vi "STORE_FREE_INPUT.vi"(9 "CURRENT_YEAR_DATA":string, 10 "ECODE 2":string, 11 "connection reference":T1) -> ()   [LabVIEW 2015]
uses:
  <vilib>/addons/database/Connection.llb/Conn ObjectReference.ctl
  Controls/ITEM_INFORMATION_CLUSTER.ctl
  Controls/ITEM_CODE_CLUSTER.ctl
  <vilib>/addons/database/Connection.llb/Conn Execute.vi
  <vilib>/addons/database/Recordset.llb/Rec Destroy - Connection.vi
  <vilib>/addons/database/_DB Variant To Data/Database Variant To Data.xnode
  <vilib>/addons/database/NI_Database_API.lvlib
  <vilib>/addons/database/Connection.llb/DB Tools Open Connec (String).vi
panel:
  in  "Store Stock":dbl
  in  "Lot Maker":string
  out "Invoice Date":timestamp format="%<%d/%m/%Y>T"
  in  "Location":string
  in  "Maker Code":string
  in  "Invoice No.":string
  in  "BUTTON_EXIT":bool
  in  "BUTTON_INPUT":bool
  in  "Unit 2":string
  in  "Quantity":dbl
  in  "Item Code":string
  in  "QR Code (F3)":string
  in  "Maker":string
  in  "Part Name":string
  in  "Product":string
  out "ECODE":string
  out "Input Date":timestamp format="%<%d/%m/%Y>T"
  in  "Input No.(F1)":string
  # "FREE INPUT"
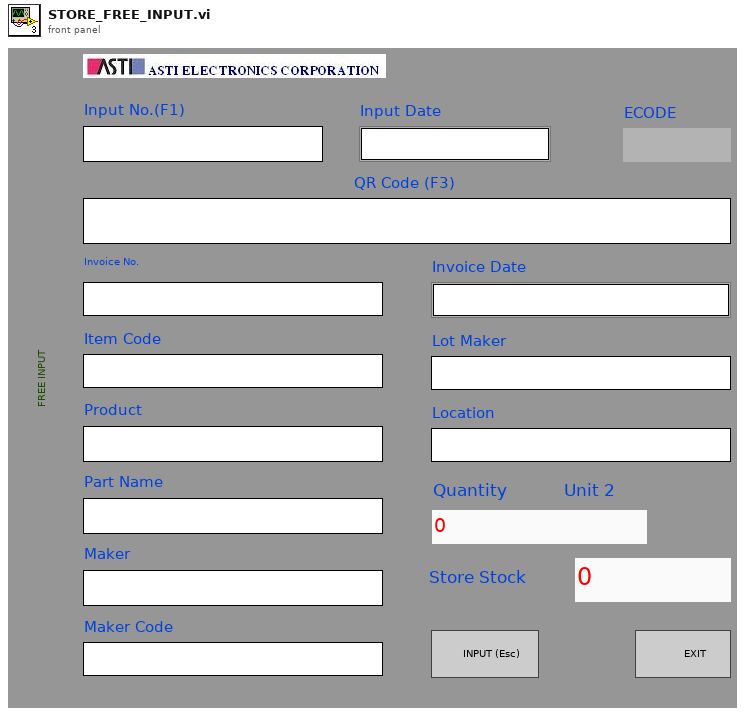
[diagram p1: front panel]
types:
  T1 = typedef "NI_Database_API.lvlib/Conn ObjectReference.ctl" = refnum<k1>
  T2 = typedef "ITEM_CODE_CLUSTER.ctl" = cluster{"ITEM_CODE":string, "INVOICE_NO":string, "INVOICE_DATE":timestamp, "LOT_MAKER":string, "QUANTITY":dbl, "INVOICE_ECODE":string, "INPUT_NO":string, "INPUT_DATE":timestamp, "INPUT_ECODE":string, "LINEBACK_NO":string, "LINEBACK_DATE":timestamp, "LINEBACK_ECODE":string, "OUTPUT_NO":string, "OUTPUT_DATE":timestamp, "OUTPUT_ECODE":string, "DESTINATION":string}
  T3 = cluster{"INVOICE_DATE":timestamp, "LOT_MAKER":string, "INVOICE_NO":string}[]
  T4 = typedef "ITEM_INFORMATION_CLUSTER.ctl" = cluster{"PRODUCT":string, "ITEM_CODE":string, "PART_NAME":string, "MAKER":string, "PART_NO":string, "LOT_SIZE":dbl, "UNIT":string, "LENGTH-OFFSET":string, "BARCODE":string, "PROCESS":string, "INVENTORY_LOCAL":string, "TARE":dbl, "SAMPLE":dbl}
  T5 = cluster{"ITEM_CODE":string, "INVOICE_NO":string, "INVOICE_DATE":timestamp, "LOT_MAKER":string, "QUANTITY":dbl, "INVOICE_ECODE":string, "INPUT_NO":string, "INPUT_DATE":timestamp, "INPUT_ECODE":string, "LINEBACK_NO":string, "LINEBACK_DATE":timestamp, "LINEBACK_ECODE":string, "OUTPUT_NO":string, "OUTPUT_DATE":timestamp, "OUTPUT_ECODE":string, "DESTINATION":string}
  T6 = cluster{"INVOICE_DATE":timestamp, "LOT_MAKER":string, "INVOICE_NO":string}
  T7 = typedef "NI_Database_API.lvlib/Rec ObjectReference.ctl" = refnum<k1>
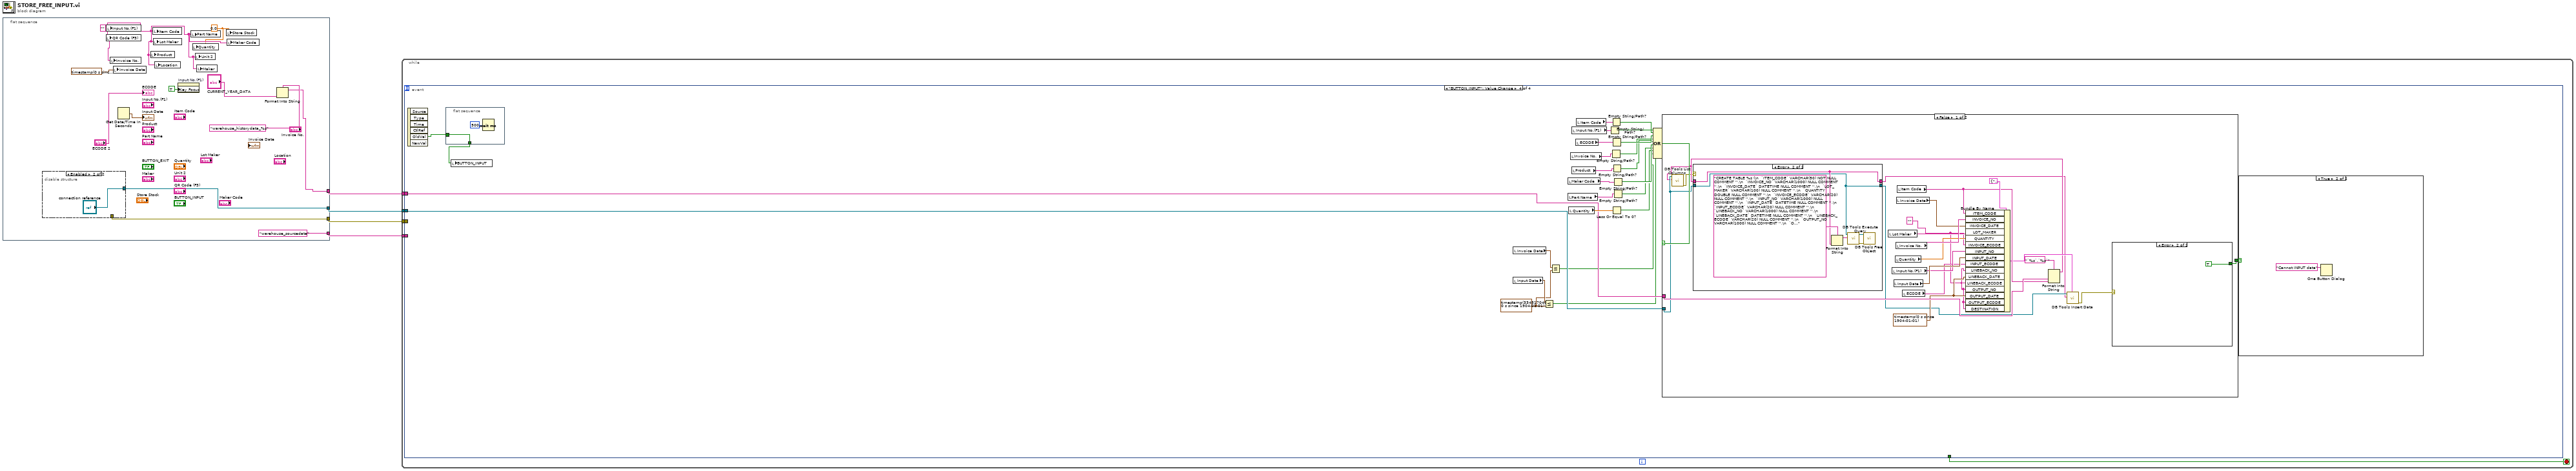
[diagram p0: block diagram]
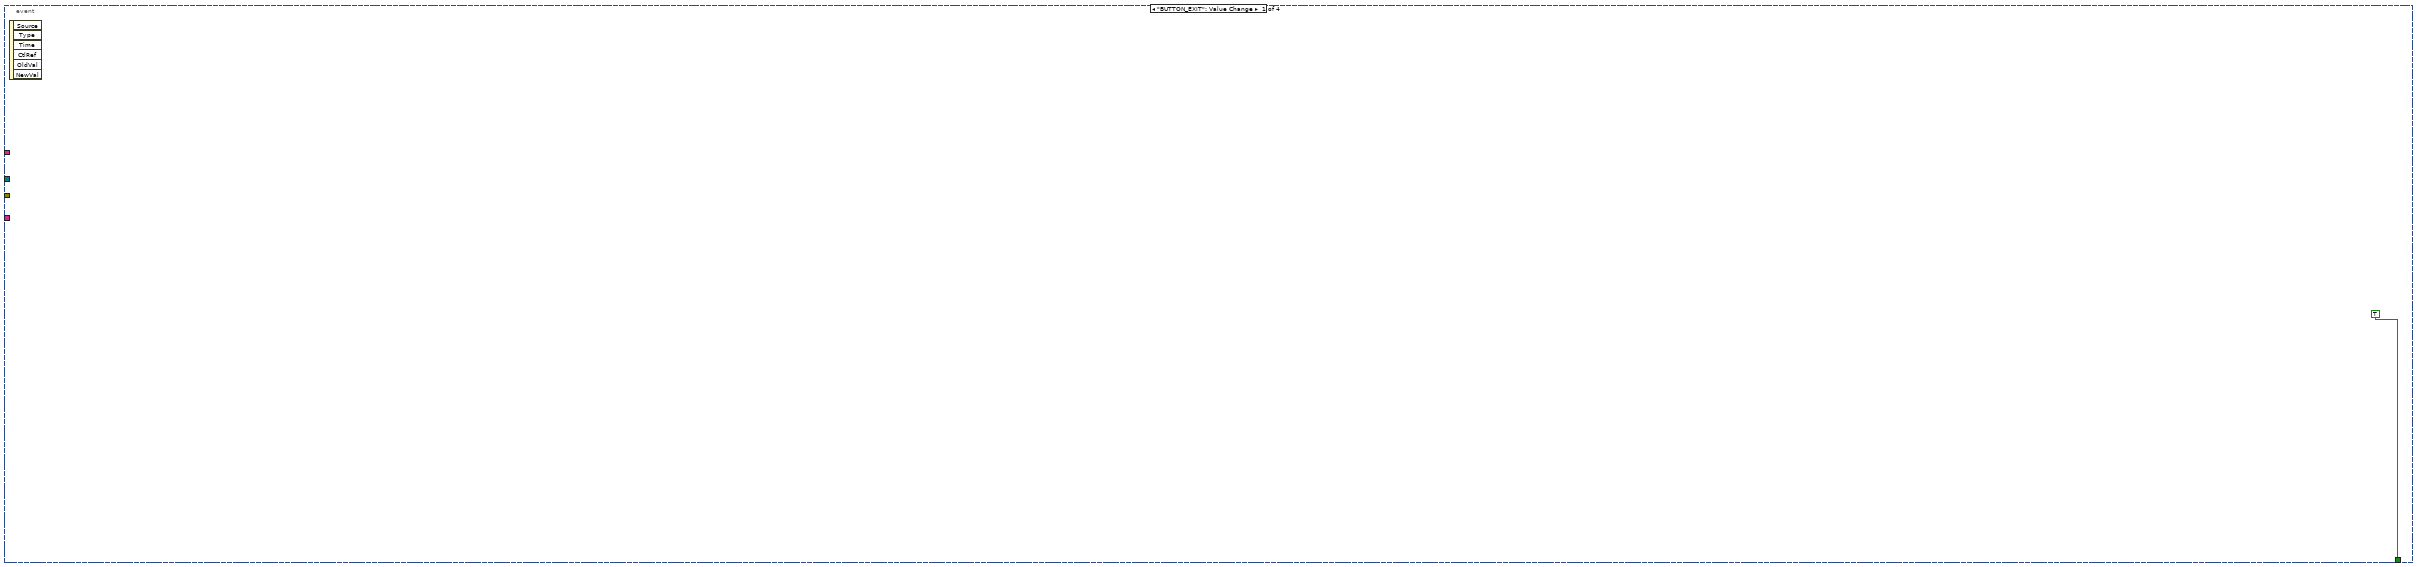
[diagram p2: hidden frame]
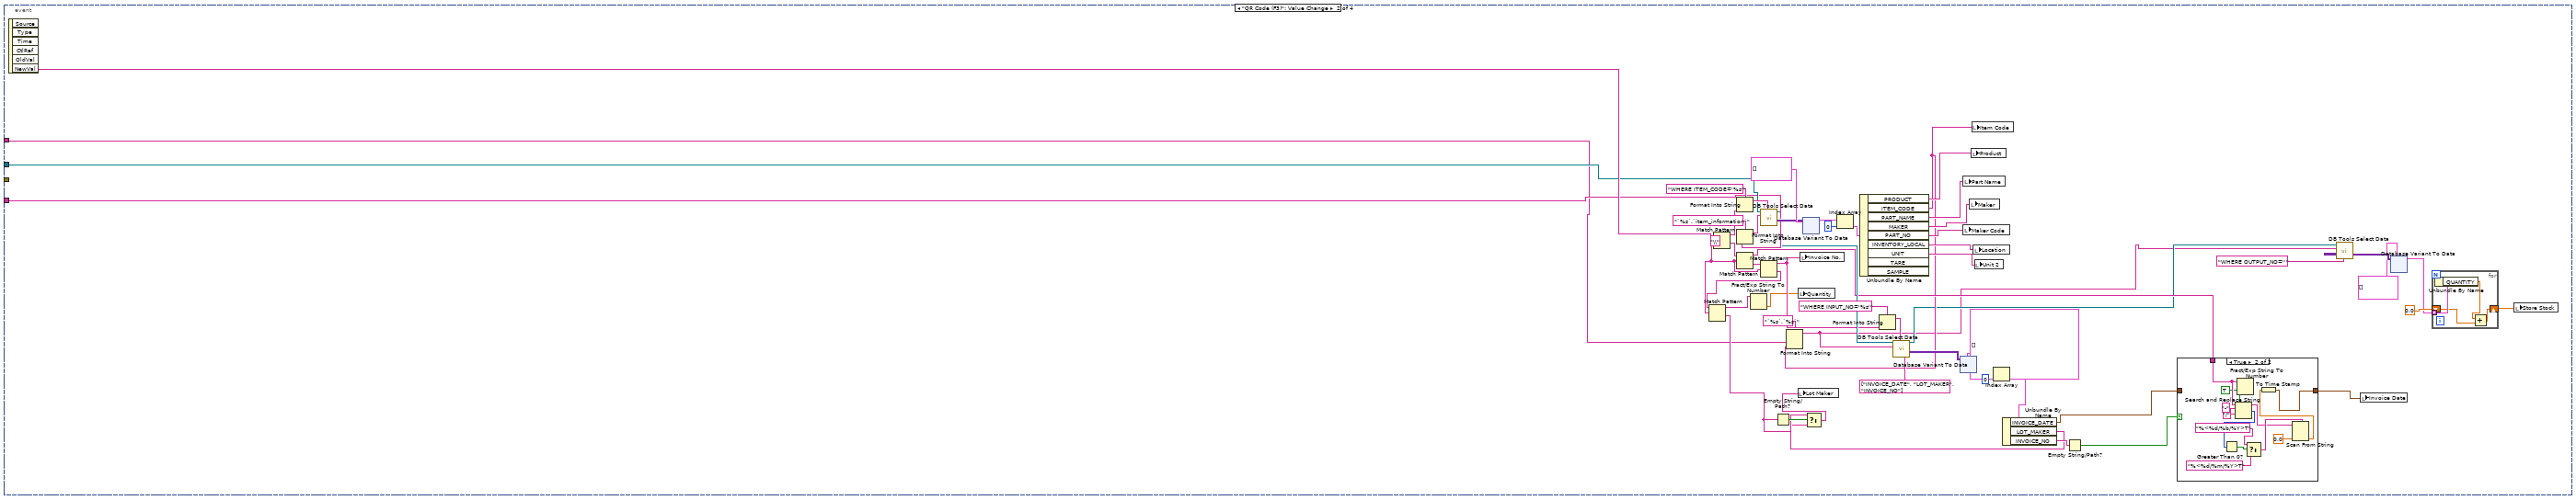
[diagram p3: hidden frame]
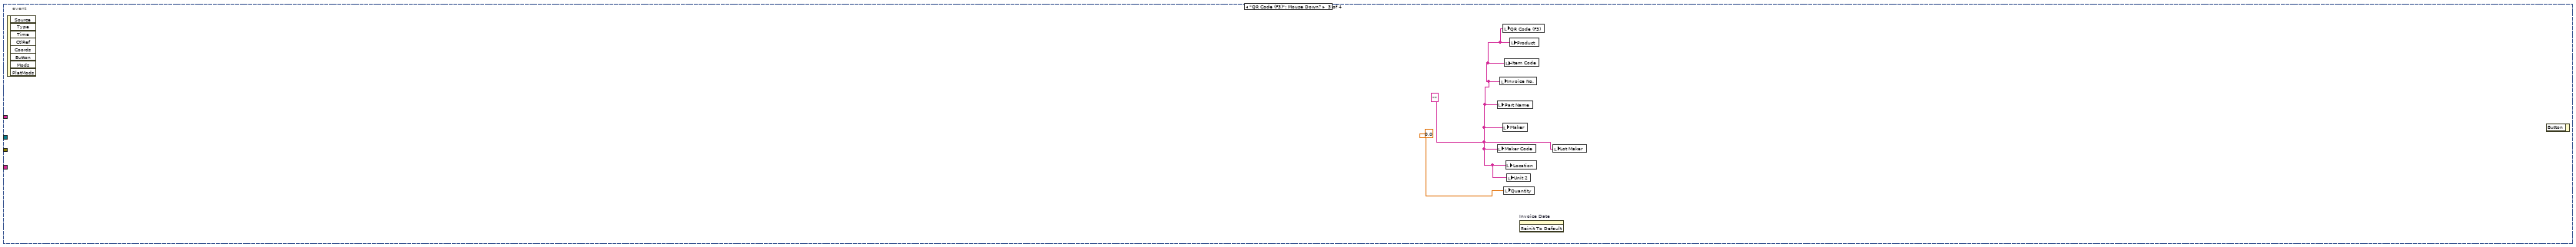
[diagram p5: hidden frame]
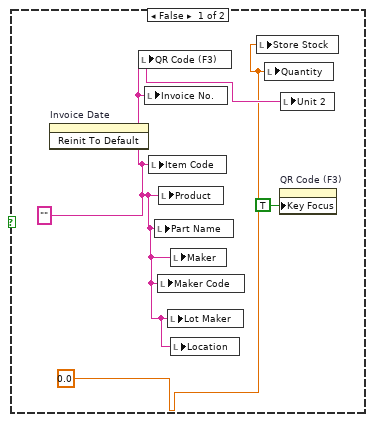
[diagram p6: hidden frame]
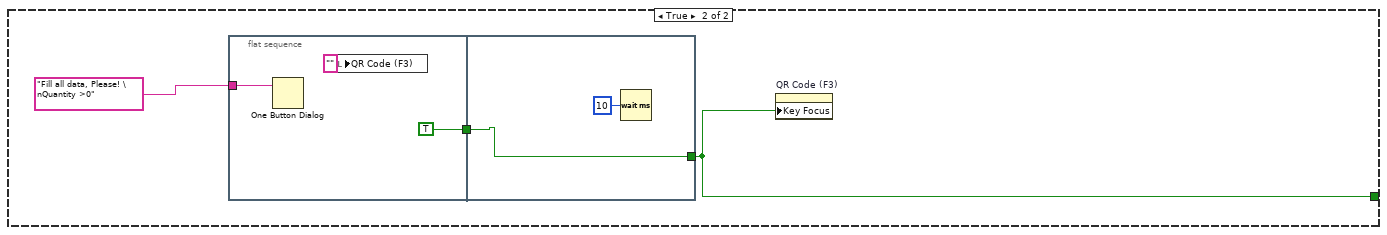
[diagram p9: hidden frame]
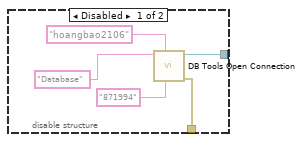
[diagram p10: hidden frame]
diagram:
  n1 = flat-sequence {
    tunnel: [w14] -> w1
    tunnel: [w13] -> w4
    tunnel: [w12] -> w3
    tunnel: ["warehouse_sourcedata" ("table")] -> w2
    frame #0 {
      w8 = 0.0 ("Store Stock")
      w9 = "" ("INPUT No.")
      n2 = disable-structure shown="Enabled" {
        disable-tunnel: [w18 "connection reference"] -> w13
        disable-tunnel: [w17 _] -> w12
        frame Disabled {
          n3 = call-poly <vilib>:"DB Tools Open Connection.vi"("password"="871994" ("userID"), "userID"="hoangbao2106", "connection information"="Database" ("userID")) -> ("error out"=w17:errorcluster, "connection reference"=w18:T1)  [unwired: 5 in]
        }
        frame Enabled {
        }
      }
      n4 = local write "QR Code (F3)"(w9) -> ()
      n5 = local write "Input No.(F1)"(w9) -> ()
      n6 = local write "Invoice No."(w9) -> ()
      n7 = local write "Invoice Date"(timestamp(0 s since 1904-01-01) ("Invoice Date")) -> ()
      n8 = Get Date/Time In Seconds() -> (seconds since 1Jan1904=→"Input Date":timestamp)
      n9 = local write "Product"(w9) -> ()
      n10 = local write "Item Code"(w9) -> ()
      n11 = local write "Lot Maker"(w9) -> ()
      n12 = local write "Location"(w9) -> ()
      n13 = property on="Input No.(F1)" class="Str"("Key Focus"=TRUE) -> ()  [unwired: 2 in, 2 out]
      n14 = local write "Part Name"(w9) -> ()
      n15 = local write "Quantity"(w8) -> ()
      n16 = local write "Unit 2"(w9) -> ()
      n17 = local write "Maker"(w9) -> ()
      n18 = local write "Store Stock"(w8) -> ()
      n19 = local write "Maker Code"(w9) -> ()
      n20 = Format Into String(format string="warehouse_historydata_%s" ("table"), "CURRENT_YEAR_DATA") -> (resulting string=w14:string)  [unwired: 2 in, 1 out]
      "ECODE" <- "ECODE 2"
    }
  }
  n21 = while {
    tunnel: w4 -> [w26]
    tunnel: w3 -> [w25]
    tunnel: w2 -> [w24]
    tunnel: w1 -> [w23]
    stop <- w27 stop-if-true
    n22 = event shown="[3] \"BUTTON_INPUT\": Value Change" {
      selector: _ -> [_ _ _ _]
      dyn-events: _ -> [_ _ _ _]
      timeout: _ -> [_ _ _ _]
      tunnel: [TRUE _ _ _] -> w27
      tunnel: w26 -> [_ w70 _ w1200]
      tunnel: w25 -> [_ _ _ _]
      tunnel: w24 -> [_ w69 _ _]
      tunnel: w23 -> [_ w32 _ w1199]
      event "BUTTON_EXIT": Value Change {
        n23 = event-data() -> ()  [unwired: 1 in, 6 out]
      }
      event "QR Code (F3)": Value Change {
        w46 = "\\" ("regular expression")
        n24 = event-data() -> ("NewVal"=w71:string)  [unwired: 1 in, 5 out]
        n25 = Match Pattern(string=w71, regular expression=w46) -> (before substring=w77:string, after substring=w72:string)  [unwired: 1 in, 2 out]
        n26 = Format Into String(format string="WHERE ITEM_CODE='%s'", w77) -> (resulting string=w78:string)  [unwired: 2 in, 1 out]
        n27 = Format Into String(format string="`%s`.`item_information`", w69) -> (resulting string=w75:string)  [unwired: 2 in, 1 out]
        n28 = Match Pattern(string=w72, regular expression=w46) -> (before substring=w50:string, after substring=w73:string)  [unwired: 1 in, 2 out]
        n29 = call <vilib>:"DB Tools Select Data.vi"("condition"=w78, "table"=w75, "connection reference"=w70) -> ("data"=w79:variant[][], "connection reference out"=w62:T1)  [unwired: 3 in, 1 out]
        n30 = Match Pattern(string=w73, regular expression=w46) -> (before substring=w59:string, after substring=w47:string)  [unwired: 1 in, 2 out]
        n31 = Match Pattern(string=w47, regular expression=w46) -> (before substring=w41:string, after substring=w42:string)  [unwired: 1 in, 2 out]
        n32 = Fract/Exp String To Number(string=w41) -> (number=w40:dbl)  [unwired: 3 in, 1 out]
        n33 = Empty String/Path?(string/path=w42) -> (empty?=w45:bool)
        n34 = local write "Quantity"(w40) -> ()
        n35 = local write "Invoice No."(w59) -> ()
        n36 = xnode "Database Variant To Data"("database variant"=w79, "type"=T4[] []) -> ("data"=w81:T4[])  [unwired: 1 in, 1 out]
        n37 = Index Array(array=w81, index=0) -> (element=w83:T4)
        n38 = Unbundle By Name(w83) -> ("PRODUCT"=w68:string, "ITEM_CODE"=w31:string, "PART_NAME"=w67:string, "MAKER"=w65:string, "PART_NO"=w66:string, "INVENTORY_LOCAL"=w64:string, "UNIT"=w63:string)  [unwired: 2 out]
        n39 = Format Into String(format string="`%s`.`%s`", w32, w31) -> (resulting string=w29:string)  [unwired: 2 in, 1 out]
        n40 = Format Into String(format string="WHERE INPUT_NO='%s'", w59) -> (resulting string=w60:string)  [unwired: 2 in, 1 out]
        n41 = call <vilib>:"DB Tools Select Data.vi"("condition"=w60, "columns"=string[] ["INVOICE_DATE", "LOT_MAKER", "INVOICE_NO"], "table"=w29, "connection reference"=w62) -> ("data"=w58:variant[][], "connection reference out"=w30:T1)  [unwired: 2 in, 1 out]
        n42 = xnode "Database Variant To Data"("database variant"=w58, "type"=T3 []) -> ("data"=w55:T3)  [unwired: 1 in, 1 out]
        n43 = local write "Part Name"(w67) -> ()
        n44 = local write "Maker Code"(w66) -> ()
        n45 = local write "Maker"(w65) -> ()
        n46 = local write "Product"(w68) -> ()
        n47 = local write "Item Code"(w31) -> ()
        n48 = local write "Location"(w64) -> ()
        n49 = local write "Unit 2"(w63) -> ()
        n50 = Index Array(array=w55, index=0 ("index (row)")) -> (element=w53:T6)
        n51 = Unbundle By Name(w53) -> ("INVOICE_DATE"=w48:timestamp, "LOT_MAKER"=w43:string, "INVOICE_NO"=w52:string)
        n52 = Select(t=w43, s=w45, f=w42) -> (s? t:f=w44:string)
        n53 = local write "Lot Maker"(w44) -> ()
        n54 = Empty String/Path?(string/path=w52) -> (empty?=w51:bool)
        n55 = case shown="True" w51 {
          tunnel: w50 -> [_ w658]
          tunnel: [w646 w659] -> w49
          tunnel: w48 -> [w646 _]
          frame False {
          }
          frame True {
            n56 = Search and Replace String(replace all?=TRUE ("replace all? (F)"), input string=w658, search string="-", replace string="/" ("replace string (\"\")")) -> (result string=w647:string, number of replacements=w654:i32)  [unwired: 4 in, 2 out]
            n57 = Greater Than 0?(x=w654) -> (x > 0?=w653:bool)
            n58 = Fract/Exp String To Number(string=w658) -> ()  [unwired: 3 in, 2 out]
            n59 = Select(t="%<%d/%b/%Y>T" ("format string"), s=w653, f="%<%d/%m/%Y>T" ("format string")) -> (s? t:f=w648:string)
            n60 = Scan From String(format string=w648, input string=w647, default 1=0.0) -> (output 1=w650:dbl)  [unwired: 2 in, 3 out]
            n61 = To Time Stamp(1:w650) -> (0:w659:timestamp)
          }
        }
        n62 = call <vilib>:"DB Tools Select Data.vi"("condition"="WHERE OUTPUT_NO=''", "table"=w29, "connection reference"=w30) -> ("data"=w35:variant[][])  [unwired: 3 in, 2 out]
        n63 = local write "Invoice Date"(w49) -> ()
        n64 = xnode "Database Variant To Data"("database variant"=w35, "type"=T2[] []) -> ("data"=w37:T2[])  [unwired: 1 in, 1 out]
        n65 = for {
          tunnel: w37 -> [w87] mode=indexing
          shift-right: [w84] -> w39
          shift-left: 0.0 -> [w85]
          n66 = Unbundle By Name(w87) -> ("QUANTITY"=w86:dbl)
          n67 = Add(x=w86, y=w85) -> (x+y=w84:dbl)
        }
        n68 = local write "Store Stock"(w39) -> ()
      }
      event "QR Code (F3)": Mouse Down? {
        w1189 = ""
        n69 = event-data() -> ()  [unwired: 1 in, 8 out]
        n70 = local write "Part Name"(w1189) -> ()
        n71 = local write "Maker Code"(w1189) -> ()
        n72 = local write "Invoice No."(w1189) -> ()
        n73 = local write "Maker"(w1189) -> ()
        n74 = local write "QR Code (F3)"(w1189) -> ()
        n75 = local write "Quantity"(0.0) -> ()
        n76 = local write "Item Code"(w1189) -> ()
        n77 = local write "Location"(w1189) -> ()
        n78 = local write "Unit 2"(w1189) -> ()
        n79 = local write "Product"(w1189) -> ()
        n80 = invoke on="Invoice Date" class="AbsTime (strict)" method="Reinit To Default"() -> ()  [unwired: 3 in, 3 out]
        n81 = local write "Lot Maker"(w1189) -> ()
        n82 = event-data() -> ()  [unwired: 2 in, 1 out]
      }
      event "BUTTON_INPUT": Value Change {
        w1196 = timestamp(3345170400 s since 1904-01-01)
        n83 = event-data() -> ("OldVal"=w1192:bool)  [unwired: 1 in, 5 out]
        n84 = flat-sequence {
          tunnel: [w1219] -> w1191
          tunnel: w1192 -> [w1219]
          frame #0 {
            n85 = Wait (ms)(milliseconds to wait=u32 500) -> ()  [unwired: 1 out]
          }
        }
        n86 = local write "BUTTON_INPUT"(w1191) -> ()
        n87 = local read "Invoice Date"() -> (w1195:timestamp)
        n88 = local read "Input Date"() -> (w1197:timestamp)
        n89 = Less Or Equal?(x=w1197, y=w1196) -> (x <= y?=w1193:bool)
        n90 = Less Or Equal?(x=w1195, y=w1196) -> (x <= y?=w1194:bool)
        n91 = local read "Maker Code"() -> (w1213:string)
        n92 = local read "Part Name"() -> (w1212:string)
        n93 = local read "Quantity"() -> (w1211:dbl)
        n94 = local read "Invoice No."() -> (w1215:string)
        n95 = local read "Product"() -> (w1214:string)
        n96 = local read "Input No.(F1)"() -> (w1217:string)
        n97 = local read "ECODE"() -> (w1216:string)
        n98 = local read "Item Code"() -> (w1202:string)
        n99 = Empty String/Path?(string/path=w1217) -> (empty?=w1210:bool)
        n100 = Empty String/Path?(string/path=w1215) -> (empty?=w1208:bool)
        n101 = Empty String/Path?(string/path=w1202) -> (empty?=w1201:bool)
        n102 = Empty String/Path?(string/path=w1216) -> (empty?=w1209:bool)
        n103 = Less Or Equal To 0?(x=w1211) -> (x <= 0?=w1204:bool)
        n104 = Empty String/Path?(string/path=w1214) -> (empty?=w1207:bool)
        n105 = Empty String/Path?(string/path=w1213) -> (empty?=w1206:bool)
        n106 = Empty String/Path?(string/path=w1212) -> (empty?=w1205:bool)
        n107 = Compound Arithmetic op=OR(w1201, w1210, w1209, w1208, w1207, w1206, w1205, w1204, w1194, w1193) -> (w1203:bool)
        n108 = case shown="False" w1203 {
          tunnel: w1200 -> [w1228 _]
          tunnel: w1199 -> [w1244 _]
          tunnel: [w1243 w1254] -> w1198
          frame False {
            w1229 = ""
            w1232 = timestamp(0 s since 1904-01-01)
            n109 = local read "Lot Maker"() -> (w1239:string)
            n110 = local read "Input No.(F1)"() -> (w1231:string)
            n111 = local read "Input Date"() -> (w1233:timestamp)
            n112 = local read "Quantity"() -> (w1238:dbl)
            n113 = local read "Invoice No."() -> (w1241:string)
            n114 = local read "Invoice Date"() -> (w1240:timestamp)
            n115 = local read "Item Code"() -> (w1236:string)
            n116 = local read "ECODE"() -> (w1230:string)
            n117 = Bundle By Name(cluster=T5 {"ITEM_CODE"="", "INVOICE_NO"="", "INVOICE_DATE"=timestamp(0 s since 1904-01-01), "LOT_MAKER"="", "QUANTITY"=0.0, "INVOICE_ECODE"="", "INPUT_NO"="", "INPUT_DATE"=timestamp(0 s since 1904-01-01), "INPUT_ECODE"="", "LINEBACK_NO"="", "LINEBACK_DATE"=timestamp(0 s since 1904-01-01), "LINEBACK_ECODE"="", "OUTPUT_NO"="", "OUTPUT_DATE"=timestamp(0 s since 1904-01-01), "OUTPUT_ECODE"="", "DESTINATION"=""}, "ITEM_CODE"=w1236, "INVOICE_NO"=w1241, "INVOICE_DATE"=w1240, "LOT_MAKER"=w1239, "QUANTITY"=w1238, "INVOICE_ECODE"=w1229, "INPUT_NO"=w1231, "INPUT_DATE"=w1233, "INPUT_ECODE"=w1230, "LINEBACK_NO"=w1229, "LINEBACK_DATE"=w1232, "LINEBACK_ECODE"=w1229, "OUTPUT_NO"=w1229, "OUTPUT_DATE"=w1232, "OUTPUT_ECODE"=w1229, "DESTINATION"=w1229) -> (w1235:T5)
            n118 = Format Into String(format string="`%s`.`%s`", w1244, w1236) -> (resulting string=w1227:string)  [unwired: 2 in, 1 out]
            n119 = call <vilib>:"DB Tools List Columns.vi"("table"=w1227, "connection reference"=w1228) -> ("error out"=w1226:errorcluster)  [unwired: 2 in, 3 out]
            n120 = case shown="Error" w1226 {
              tunnel: w1228 -> [w1246 w1247]
              tunnel: w1227 -> [w1245 w1248]
              tunnel: [w1245 w1248] -> w1224
              tunnel: [w1246 w1247] -> w1225
              frame No Error {
              }
              frame Error {
                n121 = Format Into String(format string="CREATE TABLE %s (\n  `ITEM_CODE` VARCHAR(50) NOT NULL COMMENT '',\n  `INVOICE_NO` VARCHAR(1000) NULL COMMENT '',\n  `INVOICE_DATE` DATETIME NULL COMMENT '',\n  `LOT_MAKER` VARCHAR(100) NULL COMMENT '',\n  `QUANTITY` DOUBLE NULL COMMENT '',\n  `INVOICE_ECODE` VARCHAR(20) NULL COMMENT '',\n  `INPUT_NO` VARCHAR(1000) NULL COMMENT '',\n  `INPUT_DATE` DATETIME NULL COMMENT '',\n  `INPUT_ECODE` VARCHAR(20) NULL COMMENT '',\n  `LINEBACK_NO` VARCHAR(1000) NULL COMMENT '',\n  `LINEBACK_DATE` DATETIME NULL COMMENT '',\n  `LINEBACK_ECODE` VARCHAR(20) NULL COMMENT '',\n  `OUTPUT_NO` VARCHAR(1000) NULL COMMENT '',\n  `OUTPUT_DATE` DATETIME NULL COMMENT '',\n  `OUTPUT_ECODE` VARCHAR(20) NULL COMMENT '',\n  `DESTINATION` VARCHAR(1000) NULL COMMENT '');\n", w1248) -> (resulting string=w1249:string)  [unwired: 2 in, 1 out]
                n122 = call-poly <vilib>:"DB Tools Execute Query.vi"("SQL query"=w1249, "connection reference"=w1247) -> ("error out"=w1252:errorcluster, "recordset reference"=w1251:T7)  [unwired: 6 in]
                n123 = call-poly <vilib>:"DB Tools Free Object.vi"("error in (no error)"=w1252, "recordset reference"=w1251) -> ()  [unwired: 8 in, 2 out]
              }
            }
            n124 = call <vilib>:"DB Tools Insert Data.vi"("data"=w1235, "table"=w1224, "connection reference"=w1225) -> ("error out"=w1234:errorcluster)  [unwired: 7 in, 1 out]
            n125 = case shown="Error" w1234 {
              tunnel: [_ TRUE] -> w1243
              frame No Error {
              }
              frame Error {
              }
            }
          }
          frame True {
            n126 = flat-sequence {
              tunnel: "Fill all data, Please! \nQuantity >0" ("message") -> [w1259]
              tunnel: [TRUE ("Key Focus")] -> w1256
              tunnel: w1256 -> [w1261]
              tunnel: [w1261] -> w1254
              frame #0 {
                n127 = One Button Dialog(message=w1259) -> ()  [unwired: 1 in, 1 out]
                n128 = local write "QR Code (F3)"("" ("QR Code")) -> ()
              }
              frame #1 {
                n129 = Wait (ms)(milliseconds to wait=u32 10) -> ()  [unwired: 1 out]
              }
            }
            n130 = property on="QR Code (F3)" class="Str"("Key Focus"=w1254) -> ()  [unwired: 2 in, 2 out]
          }
        }
        n131 = case shown="True" w1198 {
          frame False {
            w1222 = ""
            w1220 = 0.0
            n132 = invoke on="Invoice Date" class="AbsTime (strict)" method="Reinit To Default"() -> ()  [unwired: 3 in, 3 out]
            n133 = local write "QR Code (F3)"(w1222) -> ()
            n134 = local write "Invoice No."(w1222) -> ()
            n135 = local write "Item Code"(w1222) -> ()
            n136 = local write "Part Name"(w1222) -> ()
            n137 = local write "Maker Code"(w1222) -> ()
            n138 = local write "Product"(w1222) -> ()
            n139 = local write "Lot Maker"(w1222) -> ()
            n140 = local write "Maker"(w1222) -> ()
            n141 = local write "Location"(w1222) -> ()
            n142 = local write "Store Stock"(w1220) -> ()
            n143 = local write "Quantity"(w1220) -> ()
            n144 = property on="QR Code (F3)" class="Str"("Key Focus"=TRUE) -> ()  [unwired: 2 in, 2 out]
            n145 = local write "Unit 2"(w1222) -> ()
          }
          frame True {
            n146 = One Button Dialog(message="Cannot INPUT data") -> ()  [unwired: 1 in, 1 out]
          }
        }
      }
    }
  }
